vi "example_llm_openai_unit_test_1.vi"() -> ()   [LabVIEW 2020]
uses:
  llm_openai_chatmodels/llm_openai_chatmodels.lvclass
  message_text/message_text.lvclass
  D:/lv_llm/labview-llm-libraries/src/models/abstract_message_base/abstract_message_base.lvclass
  message_text/message.ctl
panel:
  in  "Messages":cluster{"role":string, "text":string}[](array[cluster])=[{"role"="system", "text"="Act as a math teacher and guide the student in solving the problem. You should not solve the problem. Always answer in single line."}, {"role"="user", "text"="What is x in the equation 2x + 3 = 5  ?"}]
  out "error out":errorcluster
  out "openai_key":string
  in  "model_name":string(combo)="gpt-4o-mini"
  # "1. Ensure you assign the OpenAI Key to environmental variables so it is away from the code and easy to use the examples in future.\n\n2. Use the \"Set_ENv_Var.vi\" from examples/utils folder to set the key \"labview_llm_openai_key\"."
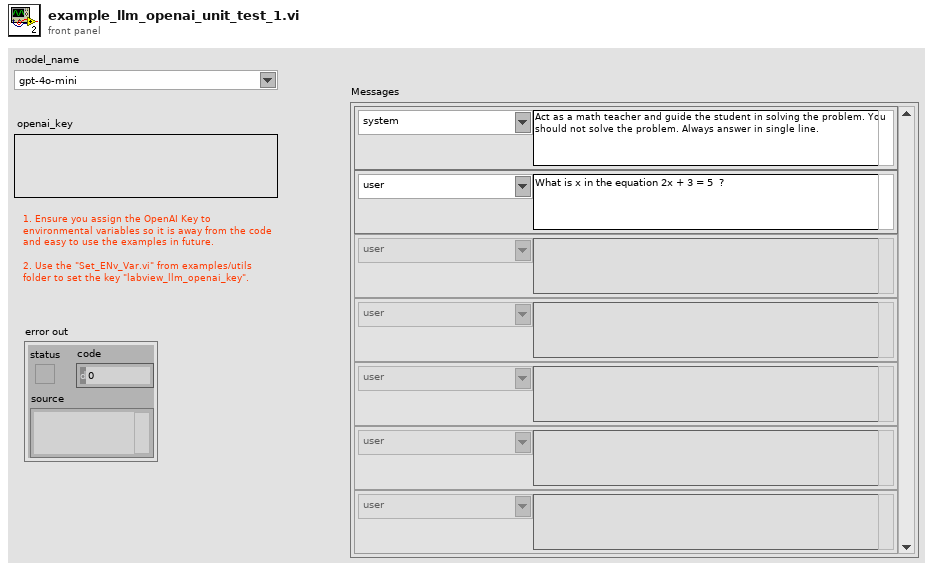
[diagram p1: front panel]
types:
  T1 = typedef "message_text.lvclass/message.ctl" = cluster{"role":string, "content":string[]}
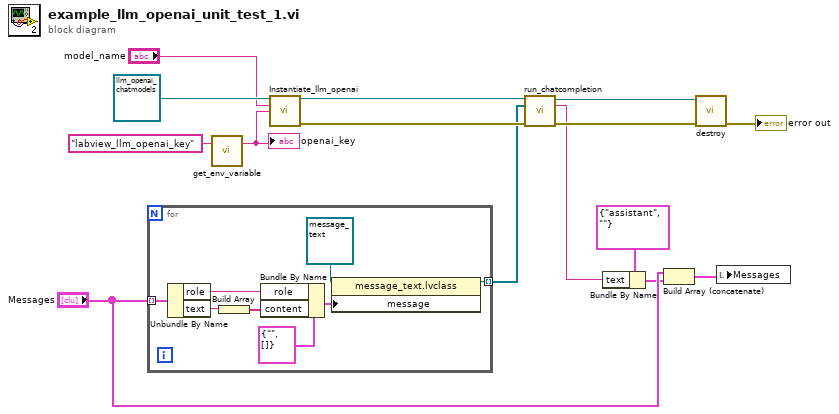
[diagram p0: block diagram]
diagram:
  n1 = for {
    tunnel: "Messages" -> [w21] mode=indexing
    tunnel: [w22] -> w6 mode=indexing
    n2 = Unbundle By Name(w21) -> ("role"=w19:string, "text"=w17:string)
    n3 = Build Array(w17) -> (w16:string[])
    n4 = Bundle By Name(cluster=T1 {"role"="", "content"=[]} ("message"), "role"=w19, "content"=w16) -> (w18:T1)
    n5 = property class="message_text.lvclass"(reference=refnum<class "message_text.lvclass"> refnum ("message_text.lvclass"), "message"=w18) -> (reference out=w22:refnum<class "message_text.lvclass">)  [unwired: 1 in, 1 out]
  }
  n6 = call "get_env_variable.vi"("Environment Variable Name"="labview_llm_openai_key") -> ("Value"=w9:string)  [unwired: 1 in, 1 out]
  "openai_key" <- w9
  n7 = call "Instantiate_llm_openai.vi"("llm_openai in"=refnum<class "llm_openai_chatmodels.lvclass"> refnum, "model_name"="model_name", "openai_key"=w9) -> ("llm_openai out"=w15:refnum<class "llm_openai_chatmodels.lvclass">, "error out"=w14:errorcluster)  [unwired: 11 in]
  n8 = call-dynamic "run_chatcompletion.vi"("chatcompletion_llm_interface in"=w15, "Messages"=w6, "error in (no error)"=w14) -> ("chatcompletion_llm_interface out"=w11:refnum<class "llm_openai_chatmodels.lvclass">, "chat response"=w2:string, "error out"=w10:errorcluster)  [unwired: 10 in]
  n9 = Bundle By Name(cluster=cluster{"role":string, "text":string} {"role"="assistant", "text"=""} ("message"), "text"=w2) -> (w1:cluster{"role":string, "text":string})
  n10 = Build Array (concatenate)("Messages", w1) -> (w4:cluster{"role":string, "text":string}[])
  n11 = call-dynamic "destroy.vi"("error in (no error)"=w10, "abstract_llm_base in"=w11) -> ("error out"=→"error out":errorcluster)  [unwired: 8 in, 1 out]
  n12 = local write "Messages"(w4) -> ()
